vi "test RT Stop.vi"(8 "error in (no error)":errorcluster, 11 "RT Stop in":refnum<class "RT Stop.lvclass">) -> (0 "error out":errorcluster, 3 "RT Stop out":refnum<class "RT Stop.lvclass">)   [LabVIEW 2016, in "RT Stop.lvclass"]
uses:
  RT Stop.lvclass
  1553 Board/1553 Board.lvclass
  PPLs/FPGA Interface.lvlibp/FPGA Interface/FPGA Interface.lvclass
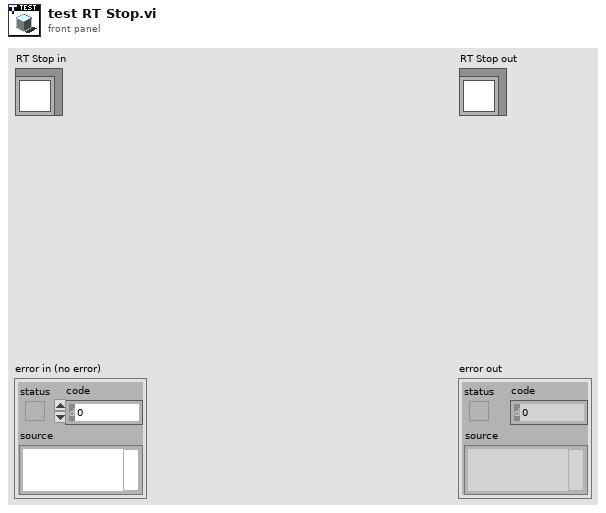
[diagram p1: front panel]
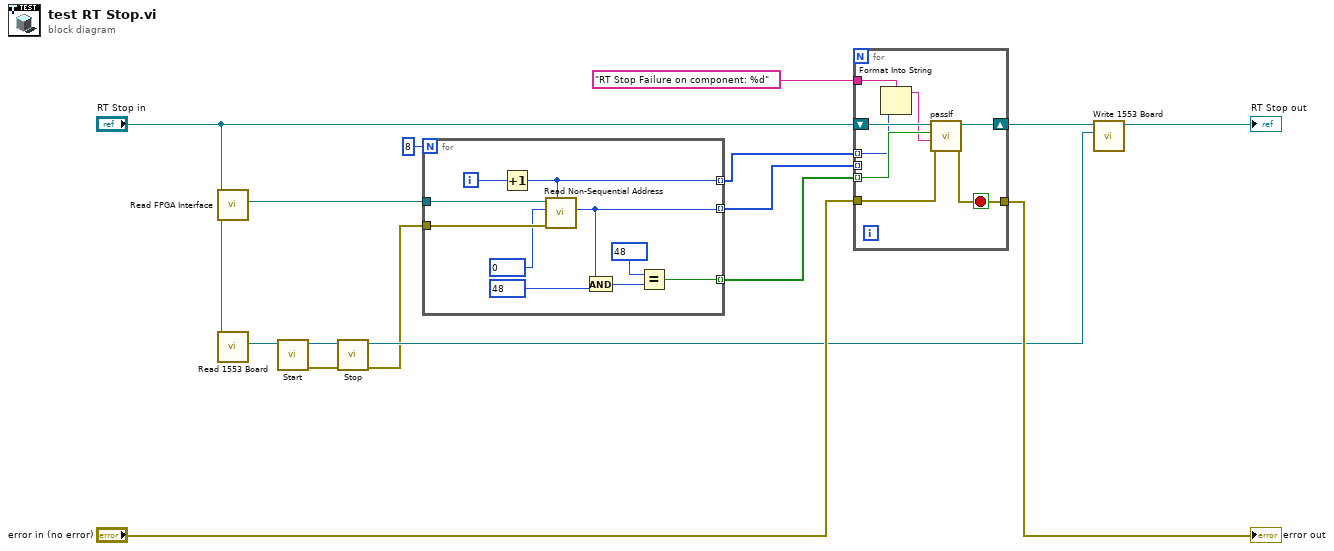
[diagram p0: block diagram]
diagram:
  n1 = call-dynamic "Read FPGA Interface.vi"("1553 Test in"="RT Stop in") -> ("FPGA Interface"=w15:refnum<class "FPGA Interface.lvclass">)  [unwired: 8 in, 2 out]
  n2 = call-dynamic "Read 1553 Board.vi"("1553 Test in"="RT Stop in") -> ("1553 Board"=w16:refnum<class "1553 Board.lvclass">)  [unwired: 8 in, 2 out]
  n3 = call-dynamic "Start.vi"("1553 Board in"=w16) -> ("error out"=w2:errorcluster, "1553 Board out"=w4:refnum<class "1553 Board.lvclass">)  [unwired: 9 in]
  n4 = call-dynamic "Stop.vi"("error in (no error)"=w2, "1553 Board in"=w4) -> ("error out"=w1:errorcluster, "1553 Board out"=w3:refnum<class "1553 Board.lvclass">)  [unwired: 8 in]
  n5 = for {
    N: 8 -> [_]
    tunnel: w15 -> [w26]
    tunnel: w1 -> [w24]
    tunnel: [w19] -> w12 mode=indexing
    tunnel: [w18] -> w11 mode=indexing
    tunnel: [w17] -> w9 mode=indexing
    i -> [w25]
    n6 = Increment(x=w25) -> (x+1=w18:i32)
    n7 = call-dynamic "Read Non-Sequential Address.vi"("Target IC (1-8)"=w18, "error in (no error)"=w24, "Address"=u16 0, "FPGA Interface in"=w26) -> ("Data"=w17:u16)  [unwired: 6 in, 1 out]
    n8 = And(x=w17, y=u16 48) -> (x .and. y?=w20:u16)
    n9 = Equal?(x=u16 48, y=w20) -> (x = y?=w19:bool)
  }
  n10 = for {
    shift-right: [w33] -> w13
    shift-left: "RT Stop in" -> [w34]
    tunnel: "error in (no error)" -> [w32]
    tunnel: [w31] -> w5
    tunnel: w12 -> [w30] mode=indexing
    tunnel: w11 -> [w28] mode=indexing
    tunnel: "RT Stop Failure on component: %d" ("custom report message (\"\")") -> [w29]
    tunnel: w9 -> [_] mode=indexing
    stop <- w31 stop-if-true
    n11 = Format Into String(format string=w29, w28) -> (resulting string=w27:string)  [unwired: 2 in, 1 out]
    n12 = call-dynamic "passIf.vi"("error in (no error)"=w32, "message (\"\")"=w27, "pass"=w30, "TestCase in"=w34) -> ("error out"=w31:errorcluster, "TestCase out"=w33:refnum<class "RT Stop.lvclass">)  [unwired: 6 in]
  }
  "error out" <- w5
  n13 = call-dynamic "Write 1553 Board.vi"("1553 Board"=w3, "1553 Test in"=w13) -> ("1553 Test out"=→"RT Stop out":refnum<class "RT Stop.lvclass">)  [unwired: 8 in, 1 out]
